vi "SIcamera_Globals.vi"() -> ()   [LabVIEW 2015]
panel:
  in  "SI Camera Manager Reference":refnum<vi>
  out "Exposure Active?":bool
  out "CCD ROI":cluster{i32, i32, i32, i32, i32, i32}={0, 4096, 1, 0, 4096, 1}
  in  "Control references":T1
  out "Start Exposure":bool
  out "Color":string
  out "Name":string
  out "Take Exp index":i32
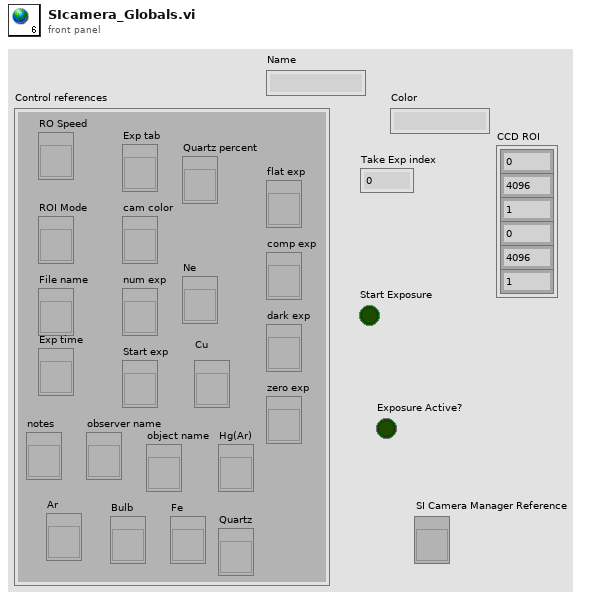
[diagram p1: front panel]
types:
  T1 = cluster{"ROI Mode":refnum<vi>, "RO Speed":refnum<vi>, "File name":refnum<vi>, "Exp time":refnum<vi>, "Start exp":refnum<vi>, "num exp":refnum<vi>, "cam color":refnum<vi>, "Exp tab":refnum<vi>, "notes":refnum<vi>, "observer name":refnum<vi>, "object name":refnum<vi>, "Ar":refnum<vi>, "Bulb":refnum<vi>, "Fe":refnum<vi>, "Hg(Ar)":refnum<vi>, "Cu":refnum<vi>, "Ne":refnum<vi>, "Quartz":refnum<vi>, "Quartz percent":refnum<vi>, "flat exp":refnum<vi>, "comp exp":refnum<vi>, "dark exp":refnum<vi>, "zero exp":refnum<vi>}
diagram:
